vi "Decrypt.vi"(8 "error in (no error)":errorcluster, 9 "Configuration":u8[](array[numeric]), 10 "IV":u8[](array[numeric]), 11 "srp":T1) -> (0 "error out":errorcluster, 2 "output":string, 3 "srp":T1)   [LabVIEW 2016, in "SRP.lvlib"]
uses:
  <vilib>/addons/InsightCM/SRP/SRP.lvlib
  <vilib>/addons/InsightCM/SRP/controls/DVR_data.ctl
  <vilib>/addons/InsightCM/SRP/controls/data.ctl
  <vilib>/addons/InsightCM/SRP/libraries/win32Urelease/brsrp.dll
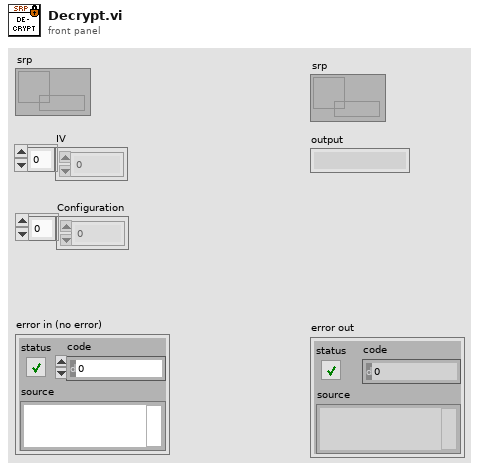
[diagram p1: front panel]
types:
  T1 = typedef "SRP.lvlib/DVR_data.ctl" = refnum<data-value>
  T2 = typedef "SRP.lvlib/data.ctl" = cluster{"SessionKey":u8[], "ClientHash":u8[], "PublicKeyA":u8[], "PrivateKeyA":u8[]}
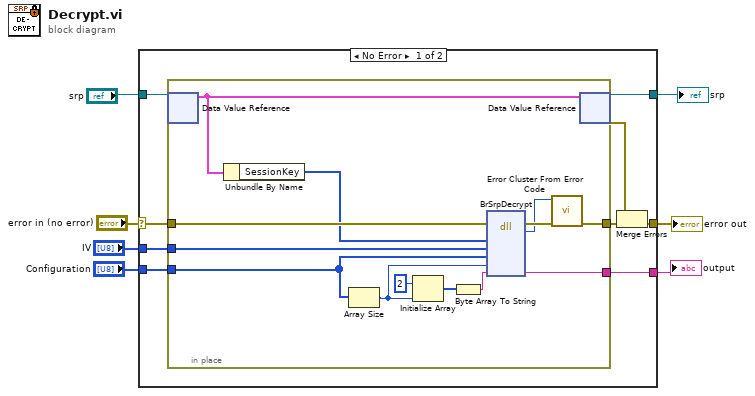
[diagram p0: block diagram]
diagram:
  n1 = case shown="No Error" "error in (no error)" {
    selector: "error in (no error)" -> [w14 w30]
    tunnel: [w16 _] -> w7
    tunnel: [w9 w30] -> w6
    tunnel: [w13 w31] -> w4
    tunnel: "srp" -> [w12 w31]
    tunnel: "Configuration" -> [w11 _]
    tunnel: "IV" -> [w10 _]
    frame No Error {
      n2 = in-place {
        in-place-border: [w24] -> w16
        in-place-border: [w23] -> w15
        in-place-border: w14 -> [w21]
        in-place-border: w11 -> [w17]
        in-place-border: w10 -> [w20]
        n3 = in-place-dvr #1(w12) -> (w19:T2)  [unwired: 1 out]
        n4 = Unbundle By Name(w19) -> ("SessionKey"=w18:u8[])
        n5 = Array Size(array=w17) -> (size(s)=w27:i32)
        n6 = Initialize Array(u8 2 ("dimension size"), w27) -> (w26:u8[])
        n7 = Byte Array To String(unsigned byte array=w26) -> (string=w25:string)
        n8 = dll-call lib="C:/Program Files (x86)/National Instruments/LabVIEW 2016/vi.lib/addons/InsightCM/SRP/libraries/win32Urelease/brsrp.*" fn="BrSrpDecrypt"(error in=w21, "key"=w18, "IV"=w20, "encrypted"=w17, "length"=w27, "output"=w25) -> (error out=w29:errorcluster, "return type"=w22:i32, "output"=w24:string)  [unwired: 6 in, 1 out]
        n9 = call <vilib>:"Error Cluster From Error Code.vi"("error in (no error)"=w29, "error code (0)"=w22) -> ("error out"=w23:errorcluster)  [unwired: 7 in]
        n10 = in-place-dvr #1(w19) -> (w13:T1, w8:errorcluster)
      }
      n11 = Merge Errors(w8, w15) -> (w9:errorcluster)
    }
    frame Error {
    }
  }
  "error out" <- w6
  "output" <- w7
  "srp" <- w4
